vi "selectHotLot.vi"() -> (0 "data":string, 2 "Array":string[][](array[string]))   [LabVIEW 2012]
uses:
  <vilib>/addons/database/Connection.llb/DB Tools Open Connec (Path).vi
  <vilib>/addons/database/_DB Variant To Data/Database Variant To Data.xnode
  <vilib>/addons/database/NI_Database_API.lvlib
panel:
  out "data 2":string
  in  "Cluster":T1
  out "error out":errorcluster
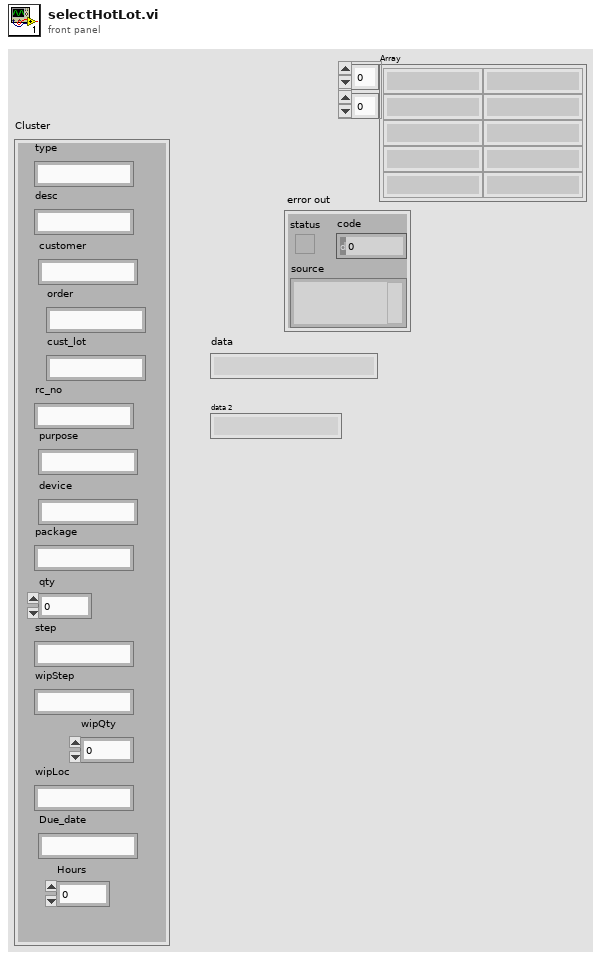
[diagram p1: front panel]
types:
  T1 = cluster{"type":string, "desc":string, "customer":string, "order":string, "cust_lot":string, "rc_no":string, "purpose":string, "device":string, "package":string, "qty":dbl, "step":string, "wipStep":string, "wipQty":dbl, "wipLoc":string, "Due_date":string, "Hours":dbl}
  T2 = typedef "NI_Database_API.lvlib/Conn ObjectReference.ctl" = refnum<k1>
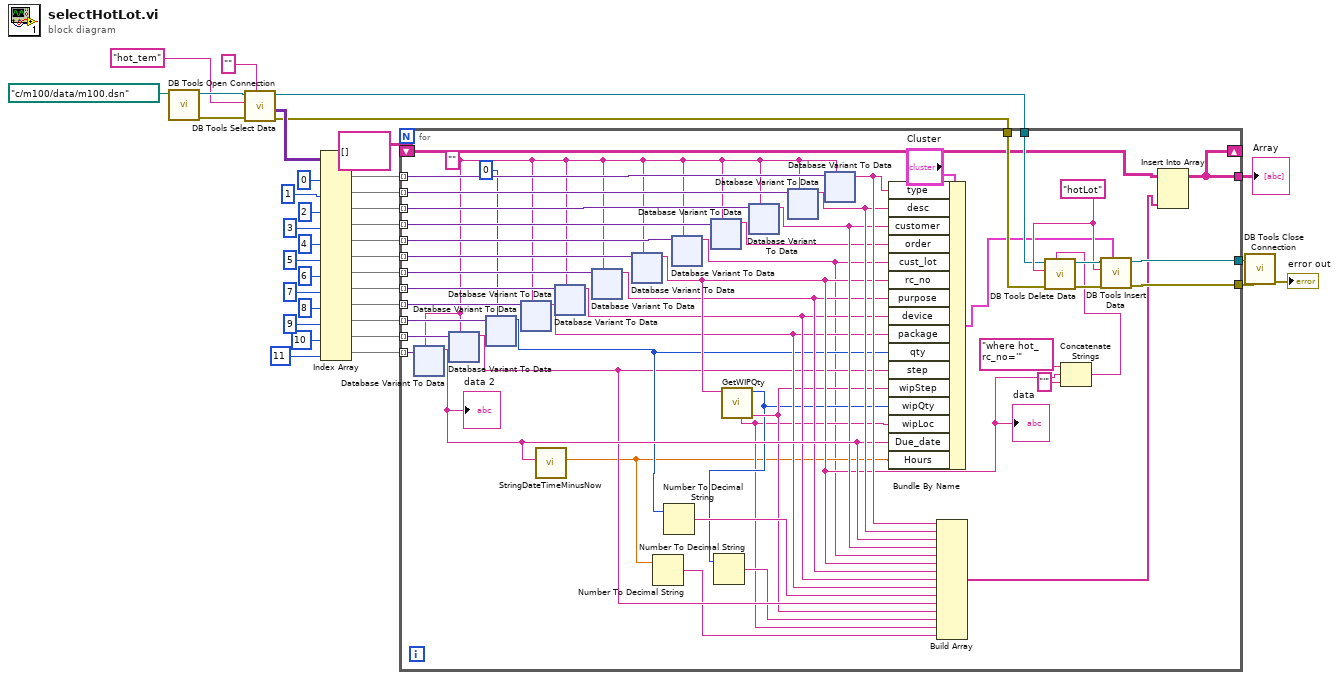
[diagram p0: block diagram]
diagram:
  n1 = call-poly <vilib>:"DB Tools Open Connection.vi"("connection information"=path "c:/m100/data/m100.dsn") -> ("error out"=w35:errorcluster, "connection reference"=w36:T2)  [unwired: 7 in]
  n2 = call <vilib>:"DB Tools Select Data.vi"("condition"="", "error in (no error)"=w35, "table"="hot_tem", "connection reference"=w36) -> ("error out"=w7:errorcluster, "data"=w20:variant[][], "connection reference out"=w8:T2)  [unwired: 2 in]
  n3 = Index Array(array=w20, index (col) #1=0 ("disabled index (col)"), index (col) #2=1 ("index (col)"), index (col) #3=2 ("index (col)"), index (col) #4=3 ("index (col)"), index (col) #5=4 ("index (col)"), index (col) #6=5 ("index (col)"), index (col) #7=6 ("index (col)"), index (col) #8=7 ("index (col)"), index (col) #9=8 ("index (col)"), index (col) #10=9 ("index (col)"), index (col) #11=10 ("index (col)"), index (col) #12=11 ("index (col)")) -> (element #1=w19:variant[], element #2=w18:variant[], element #3=w17:variant[], element #4=w16:variant[], element #5=w15:variant[], element #6=w14:variant[], element #7=w13:variant[], element #8=w12:variant[], element #9=w11:variant[], element #10=w10:variant[], element #11=w9:variant[], element #12=w3:variant[])  [unwired: 12 in]
  n4 = for {
    tunnel: w19 -> [w85] mode=indexing
    tunnel: w18 -> [w84] mode=indexing
    tunnel: w17 -> [w83] mode=indexing
    tunnel: w16 -> [w82] mode=indexing
    tunnel: w15 -> [w81] mode=indexing
    tunnel: w14 -> [w80] mode=indexing
    tunnel: w13 -> [w79] mode=indexing
    tunnel: w12 -> [w78] mode=indexing
    tunnel: w11 -> [w77] mode=indexing
    tunnel: w10 -> [w75] mode=indexing
    tunnel: w9 -> [w76] mode=indexing
    tunnel: w8 -> [w66]
    tunnel: w7 -> [w67]
    tunnel: [w72] -> w6
    tunnel: [w71] -> w5
    tunnel: w3 -> [w62] mode=indexing
    shift-right: [w58] -> _
    shift-left: string[][] [] -> [w59]
    tunnel: [w58] -> w1
    w68 = "hotLot" ("table")
    w61 = ""
    n5 = xnode "Database Variant To Data"("database variant"=w62, "type"=w61) -> ("data"=w55:string)  [unwired: 1 in, 1 out]
    "data 2" <- w55
    n6 = xnode "Database Variant To Data"("database variant"=w76, "type"=w61) -> ("data"=w46:string)  [unwired: 1 in, 1 out]
    n7 = xnode "Database Variant To Data"("database variant"=w75, "type"=0) -> ("data"=w48:i32)  [unwired: 1 in, 1 out]
    n8 = xnode "Database Variant To Data"("database variant"=w77, "type"=w61) -> ("data"=w49:string)  [unwired: 1 in, 1 out]
    n9 = call "StringDateTimeMinusNow.vi"("String DateTime"=w55) -> ("DateTime - Now"=w41:dbl)  [unwired: 10 in]
    n10 = xnode "Database Variant To Data"("database variant"=w78, "type"=w61) -> ("data"=w50:string)  [unwired: 1 in, 1 out]
    n11 = xnode "Database Variant To Data"("database variant"=w79, "type"=w61) -> ("data"=w51:string)  [unwired: 1 in, 1 out]
    n12 = xnode "Database Variant To Data"("database variant"=w80, "type"=w61) -> ("data"=w52:string)  [unwired: 1 in, 1 out]
    "data" <- w52
    n13 = Number To Decimal String(number=w41) -> (decimal integer string=w40:string)  [unwired: 1 in]
    n14 = Number To Decimal String(number=w48) -> (decimal integer string=w47:string)  [unwired: 1 in]
    n15 = xnode "Database Variant To Data"("database variant"=w81, "type"=w61) -> ("data"=w38:string)  [unwired: 1 in, 1 out]
    n16 = xnode "Database Variant To Data"("database variant"=w82, "type"=w61) -> ("data"=w53:string)  [unwired: 1 in, 1 out]
    n17 = call "GetWIPQty.vi"("Lotno"=w52) -> ("step"=w45:string, "data"=w44:i32, "location"=w42:string)  [unwired: 6 in, 2 out]
    n18 = Number To Decimal String(number=w44) -> (decimal integer string=w43:string)  [unwired: 1 in]
    n19 = xnode "Database Variant To Data"("database variant"=w83, "type"=w61) -> ("data"=w54:string)  [unwired: 1 in, 1 out]
    n20 = xnode "Database Variant To Data"("database variant"=w84, "type"=w61) -> ("data"=w56:string)  [unwired: 1 in, 1 out]
    n21 = xnode "Database Variant To Data"("database variant"=w85, "type"=w61) -> ("data"=w57:string)  [unwired: 1 in, 1 out]
    n22 = Bundle By Name(cluster="Cluster", "type"=w57, "desc"=w56, "customer"=w54, "order"=w53, "cust_lot"=w38, "rc_no"=w52, "purpose"=w51, "device"=w50, "package"=w49, "qty"=w48, "step"=w46, "wipStep"=w45, "wipQty"=w44, "wipLoc"=w42, "Due_date"=w55, "Hours"=w41) -> (w60:T1)
    n23 = Build Array(w57, w56, w55, w54, w38, w52, w51, w50, w49, w47, w46, w45, w43, w42, w40) -> (w39:string[])
    n24 = Concatenate Strings("where hot_rc_no='" ("string"), w52, "'" ("string")) -> (w63:string)
    n25 = call <vilib>:"DB Tools Delete Data.vi"("condition"=w63, "error in (no error)"=w67, "table"=w68, "connection reference"=w66) -> ("error out"=w69:errorcluster, "connection reference out"=w70:T2)  [unwired: 6 in]
    n26 = call <vilib>:"DB Tools Insert Data.vi"("data"=w60, "error in (no error)"=w69, "table"=w68, "connection reference"=w70) -> ("error out"=w71:errorcluster, "connection reference out"=w72:T2)  [unwired: 6 in]
    n27 = Insert Into Array(array=w59, new element=w39) -> (w58:string[][])  [unwired: 2 in]
  }
  "Array" <- w1
  n28 = call <vilib>:"DB Tools Close Connection.vi"("error in (no error)"=w5, "connection reference"=w6) -> ("error out"=→"error out":errorcluster)  [unwired: 5 in]
